vi "Z Go.vi"(4 "Increment":bool, 6 "Return Immediately":bool, 8 "error in (no error)":errorcluster, 9 "Speed In":dbl format="%#_13g", 10 "Position In":dbl format="%#_13g", 11 "Gantry In":refnum<k24>) -> (0 "error out":errorcluster, 1 "Speed Out":dbl, 2 "Position Out":dbl, 3 "Gantry Out":refnum<k24>)   [LabVIEW 2021, in "A3200.lvclass"]
uses:
  A3200.lvclass
  C:/Program Files (x86)/Aerotech/A3200/LabVIEW/2010/Bin/Aerotech.A3200.dll
  Program Files (x86)/Aerotech/A3200/LabVIEW/2010/Bin/Aerotech.A3200.dll
  Drivers/Aerotech A3200/Motion/MoveIncSingle.vi
  A3200.lvclass/A3200.ctl
  Drivers/Aerotech A3200/Aerotech.lvlib
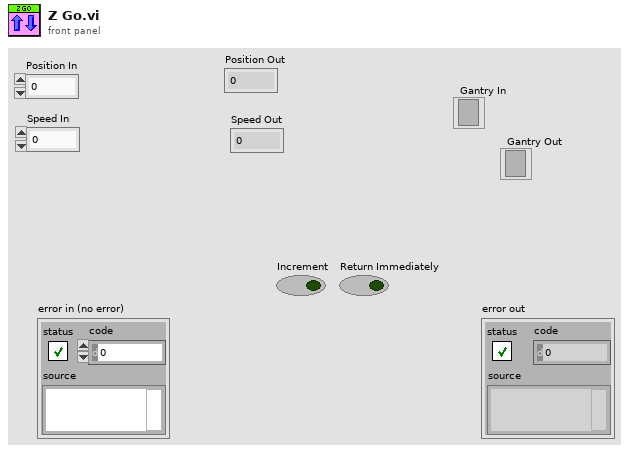
[diagram p1: front panel]
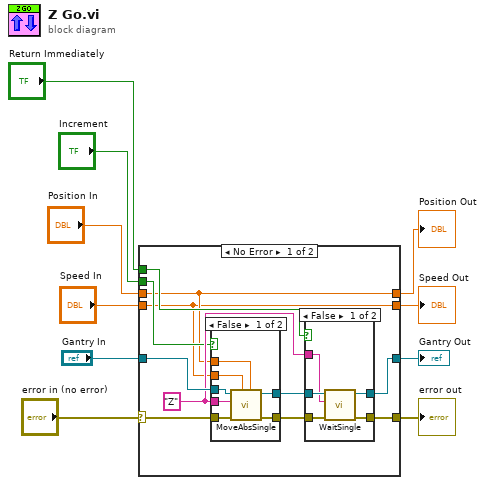
[diagram p0: block diagram]
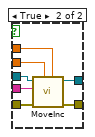
[diagram p3: hidden frame]
diagram:
  n1 = case shown="No Error" "error in (no error)" {
    selector: "error in (no error)" -> [w17 w46]
    tunnel: [w15 w46] -> w9
    tunnel: "Gantry In" -> [w20 w45]
    tunnel: [w21 w45] -> w7
    tunnel: "Increment" -> [w14 _]
    tunnel: "Return Immediately" -> [w13 _]
    tunnel: [w11 w43] -> w4
    tunnel: [w12 w44] -> w3
    tunnel: "Position In" -> [w12 w44]
    tunnel: "Speed In" -> [w11 w43]
    frame No Error {
      w18 = "Z"
      n2 = case shown="False" w14 {
        tunnel: w20 -> [w35 w42]
        tunnel: w11 -> [w30 w41]
        tunnel: w12 -> [w29 w40]
        tunnel: [w34 w39] -> w19
        tunnel: w18 -> [w33 w38]
        tunnel: w17 -> [w32 w37]
        tunnel: [w31 w36] -> w16
        frame False {
          n3 = call "MoveAbsSingle.vi"("position"=w29, "speed"=w30, "error in (no error)"=w32, "axis name"=w33, "controller in"=w35) -> ("error out"=w31:errorcluster, "controller out"=w34:refnum<k24>)  [unwired: 5 in]
        }
        frame True {
          n4 = call-poly "MoveInc.vi"("distance"=w40, "speed"=w41, "error in (no error)"=w37, "axis name"=w38, "controller in"=w42) -> ("error out"=w36:errorcluster, "controller out"=w39:refnum<k24>)  [unwired: 5 in]
        }
      }
      n5 = case shown="False" w13 {
        tunnel: [w26 w28] -> w21
        tunnel: w19 -> [w25 w28]
        tunnel: w18 -> [w24 _]
        tunnel: w16 -> [w23 w27]
        tunnel: [w22 w27] -> w15
        frame False {
          n6 = call "WaitSingle.vi"("error in (no error)"=w23, "axis name"=w24, "controller in"=w25) -> ("error out"=w22:errorcluster, "controller out"=w26:refnum<k24>)  [unwired: 6 in, 1 out]
        }
        frame True {
        }
      }
    }
    frame Error {
    }
  }
  "error out" <- w9
  "Gantry Out" <- w7
  "Speed Out" <- w4
  "Position Out" <- w3
